vi "Script Cases.vi"(0 "primitive":i32, 1 "argument 1":dbl, 2 "argument 2":dbl, 3 "argument 3":dbl, 4 "argument 4":dbl, 5 "argument 5":dbl) -> ()   [LabVIEW 2014]
uses:
  Begin/Global Variables.vi
  Begin/Global RefNums.vi
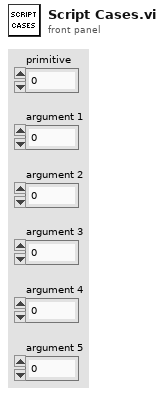
[diagram p1: front panel]
types:
  T1 = typedef "WPI_CounterDevRef.ctl" = cluster{"DevStatus":errorcluster, "CntIndex":T2}
  T2 = typedef "FPGA_CounterCtrSystemIndex.ctl" = enum8{"Ctr 0", "Ctr 1", "Ctr 2", "Ctr 3", "Ctr 4", "Ctr 5", "Ctr 6", "Ctr 7", "Invalid"}
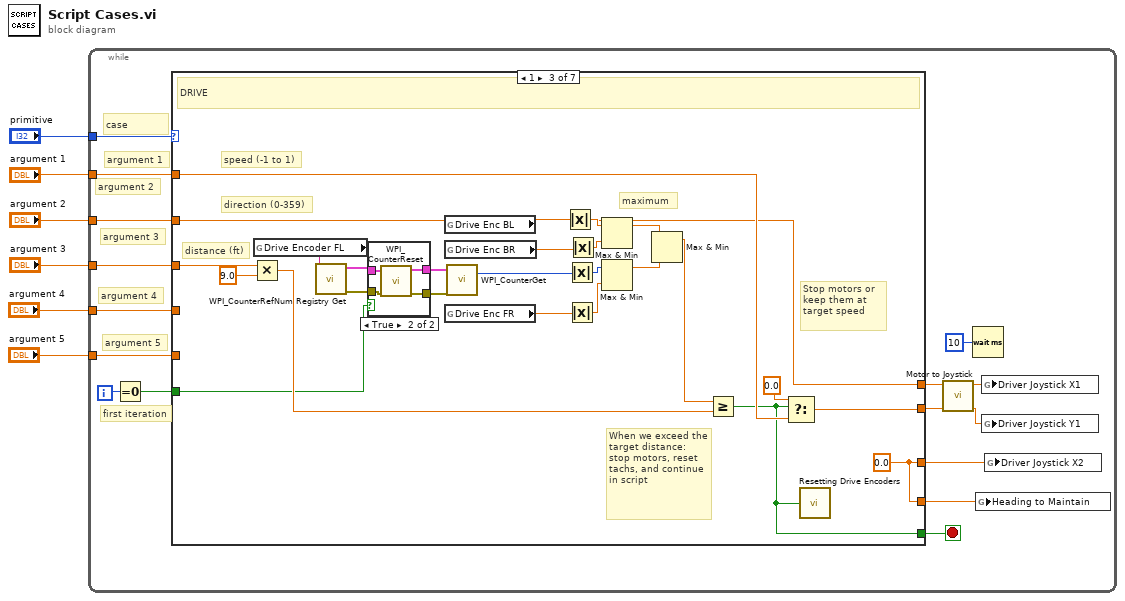
[diagram p0: block diagram]
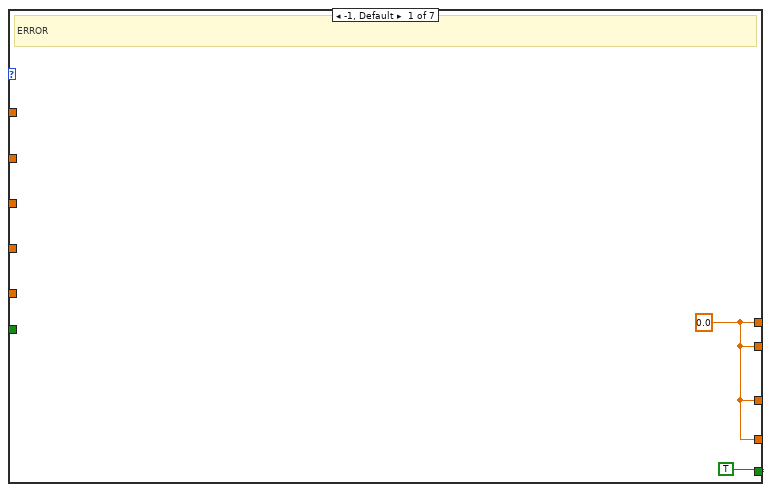
[diagram p2: hidden frame]
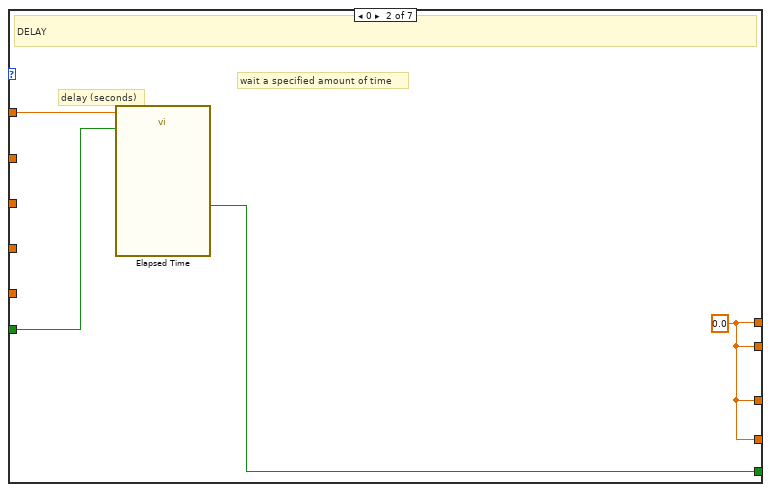
[diagram p3: hidden frame]
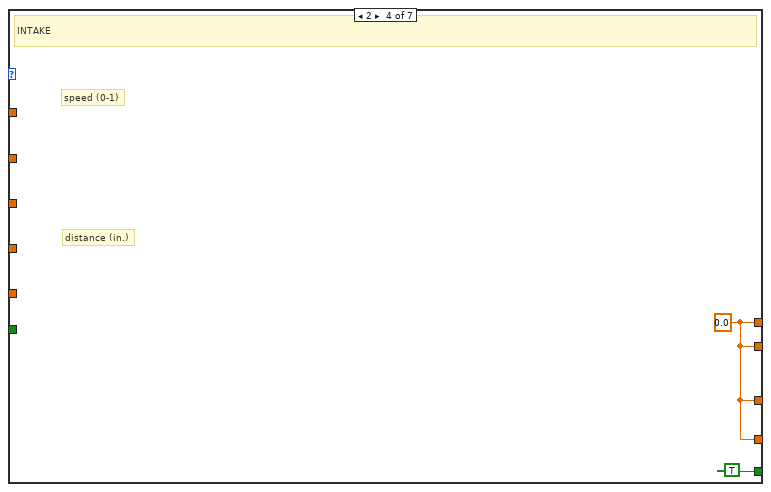
[diagram p5: hidden frame]
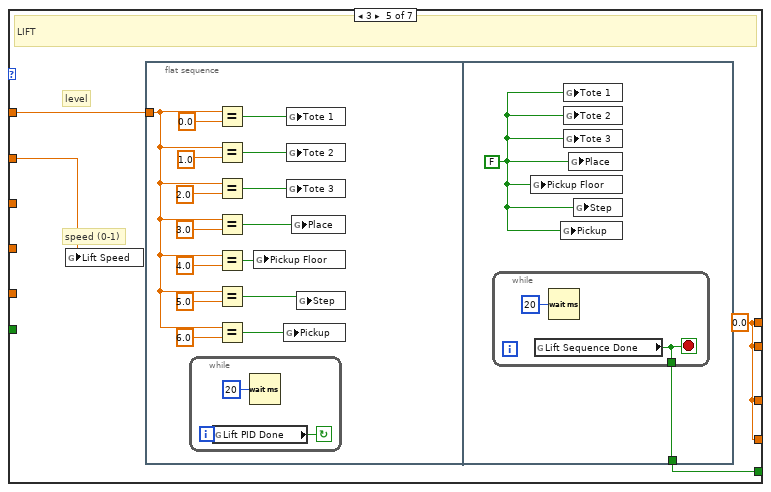
[diagram p6: hidden frame]
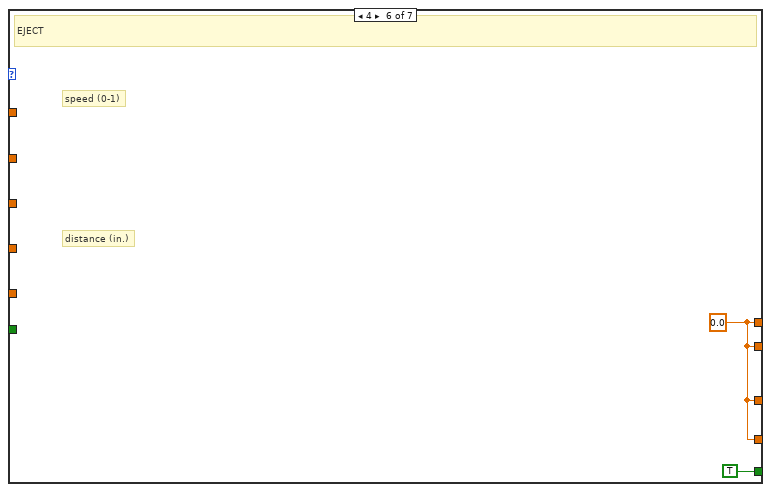
[diagram p7: hidden frame]
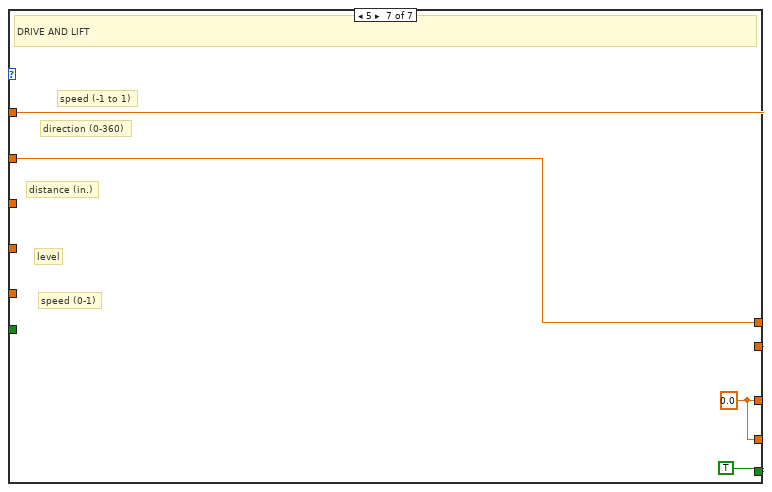
[diagram p8: hidden frame]
diagram:
  n1 = while {
    tunnel: "argument 1" -> [w22]
    tunnel: "argument 2" -> [w21]
    tunnel: "argument 3" -> [w20]
    tunnel: "argument 4" -> [w19]
    tunnel: "argument 5" -> [w18]
    tunnel: "primitive" -> [w17]
    i -> [w15]
    stop <- w16 stop-if-true
    # "first iteration"
    # "case"
    # "argument 5"
    # "argument 4"
    # "argument 3"
    # "argument 2"
    # "argument 1"
    n2 = Equal To 0?(x=w15) -> (x = 0?=w14:bool)
    n3 = case shown="1" w17 {
      tunnel: w22 -> [_ w28 w54 _ w65 _ w92]
      tunnel: w21 -> [_ _ w30 _ w66 _ w91]
      tunnel: w20 -> [_ _ w52 _ _ _ _]
      tunnel: w19 -> [_ _ _ _ _ _ _]
      tunnel: w18 -> [_ _ _ _ _ _ _]
      tunnel: [TRUE w26 w41 TRUE w63 TRUE TRUE] -> w16
      tunnel: w14 -> [_ w27 w34 _ _ _ _]
      tunnel: [w23 w25 w46 w61 w64 w88 w92] -> w11
      tunnel: [w23 w25 w30 w61 w64 w88 w91] -> w10
      tunnel: [w23 w25 w29 w61 w64 w88 w90] -> w9
      tunnel: [w23 w25 w29 w61 w64 w88 w90] -> w8
      frame -1, Default {
        w23 = 0.0 ("argument 1")
        # "ERROR"
      }
      frame 0 {
        w25 = 0.0 ("argument 1")
        # "wait a specified amount of time"
        # "delay (seconds)"
        # "DELAY"
        n4 = call "Elapsed Time"("Time Target (s)"=w28, "Reset"=w27) -> ("Time has Elapsed"=w26:bool)  [unwired: 10 in, 7 out]
      }
      frame 1 {
        w29 = 0.0 ("argument 1")
        # "When we exceed the target distance: stop motors, reset tachs, and continue in script"
        # "maximum"
        # "Stop motors or keep them at target speed"
        # "distance (ft)"
        # "direction (0-359)"
        # "speed (-1 to 1)"
        # "DRIVE"
        n5 = Multiply(x=w52, y=9.0) -> (x*y=w50:dbl)
        n6 = global read "Global RefNums.vi" "Drive Encoder FL"() -> (w35:string)
        n7 = call <vilib>:"WPI_CounterRefNum Registry Get.vi"("refnum name"=w35) -> ("error out"=w31:errorcluster, "CounterDevRef"=w32:T1)  [unwired: 9 in]
        n8 = case shown="True" w34 {
          tunnel: w32 -> [w56 w60]
          tunnel: w31 -> [w55 w59]
          tunnel: [w56 w58] -> w37
          tunnel: [w55 w57] -> w36
          frame False {
          }
          frame True {
            n9 = call <vilib>:"WPI_CounterReset.vi"("error in (no error)"=w59, "CounterDevRef in"=w60) -> ("error out"=w57:errorcluster, "CounterDevRef out"=w58:T1)  [unwired: 8 in]
          }
        }
        n10 = global read "Global Variables.vi" "Drive Enc BL"() -> (w40:dbl)
        n11 = global read "Global Variables.vi" "Drive Enc BR"() -> (w39:dbl)
        n12 = global read "Global Variables.vi" "Drive Enc FR"() -> (w38:dbl)
        n13 = call <vilib>:"WPI_CounterGet.vi"("error in (no error)"=w36, "CounterDevRef in"=w37) -> ("Value"=w33:i32)  [unwired: 4 in, 5 out]
        n14 = Absolute Value(x=w40) -> (abs(x)=w42:dbl)
        n15 = Absolute Value(x=w33) -> (abs(x)=w44:i32)
        n16 = Absolute Value(x=w38) -> (abs(x)=w43:dbl)
        n17 = Absolute Value(x=w39) -> (abs(x)=w45:dbl)
        n18 = Max & Min(x=w42, y=w45) -> (max(x,y)=w49:dbl)  [unwired: 1 out]
        n19 = Max & Min(x=w44, y=w43) -> (max(x,y)=w48:dbl)  [unwired: 1 out]
        n20 = Max & Min(x=w49, y=w48) -> (max(x,y)=w47:dbl)  [unwired: 1 out]
        n21 = Greater Or Equal?(x=w47, y=w50) -> (x >= y?=w41:bool)
        n22 = Select(t=0.0, s=w41, f=w54) -> (s? t:f=w46:dbl)
        n23 = call "Resetting Drive Encoders.vi"("Reset Encoders"=w41) -> ()  [unwired: 1 in]
      }
      frame 2 {
        w61 = 0.0 ("argument 1")
        # "distance (in.)"
        # "speed (0-1)"
        # "INTAKE"
      }
      frame 3 {
        w64 = 0.0 ("argument 1")
        # "speed (0-1)"
        # "level"
        # "LIFT"
        n24 = global write "Global Variables.vi" "Lift Speed"(w66) -> ()
        n25 = flat-sequence {
          tunnel: w65 -> [w68]
          tunnel: [w84] -> w63
          frame #0 {
            n26 = while {
              stop <- w82 continue-if-true
              n27 = global read "Global Variables.vi" "Lift PID Done"() -> (w82:bool)
              n28 = Wait (ms)(milliseconds to wait=u32 20) -> ()  [unwired: 1 out]
            }
            n29 = Equal?(x=w68, y=0.0 ("x")) -> (x = y?=w80:bool)
            n30 = Equal?(x=w68, y=1.0 ("x")) -> (x = y?=w79:bool)
            n31 = Equal?(x=w68, y=2.0 ("x")) -> (x = y?=w81:bool)
            n32 = Equal?(x=w68, y=3.0) -> (x = y?=w78:bool)
            n33 = Equal?(x=w68, y=4.0) -> (x = y?=w77:bool)
            n34 = Equal?(x=w68, y=5.0) -> (x = y?=w73:bool)
            n35 = Equal?(x=w68, y=6.0) -> (x = y?=w72:bool)
            n36 = global write "Global Variables.vi" "Pickup Floor"(w77) -> ()
            n37 = global write "Global Variables.vi" "Pickup"(w72) -> ()
            n38 = global write "Global Variables.vi" "Tote 1"(w80) -> ()
            n39 = global write "Global Variables.vi" "Tote 2"(w79) -> ()
            n40 = global write "Global Variables.vi" "Tote 3"(w81) -> ()
            n41 = global write "Global Variables.vi" "Place"(w78) -> ()
            n42 = global write "Global Variables.vi" "Step"(w73) -> ()
          }
          frame #1 {
            w85 = FALSE ("Tote 0")
            n43 = while {
              tunnel: [w86] -> w84
              stop <- w86 stop-if-true
              n44 = global read "Global Variables.vi" "Lift Sequence Done"() -> (w86:bool)
              n45 = Wait (ms)(milliseconds to wait=u32 20) -> ()  [unwired: 1 out]
            }
            n46 = global write "Global Variables.vi" "Pickup Floor"(w85) -> ()
            n47 = global write "Global Variables.vi" "Pickup"(w85) -> ()
            n48 = global write "Global Variables.vi" "Tote 1"(w85) -> ()
            n49 = global write "Global Variables.vi" "Tote 2"(w85) -> ()
            n50 = global write "Global Variables.vi" "Tote 3"(w85) -> ()
            n51 = global write "Global Variables.vi" "Place"(w85) -> ()
            n52 = global write "Global Variables.vi" "Step"(w85) -> ()
          }
        }
      }
      frame 4 {
        w88 = 0.0 ("argument 1")
        # "distance (in.)"
        # "speed (0-1)"
        # "EJECT"
      }
      frame 5 {
        w90 = 0.0 ("argument 1")
        # "speed (0-1)"
        # "level"
        # "distance (in.)"
        # "direction (0-360)"
        # "speed (-1 to 1)"
        # "DRIVE AND LIFT"
      }
    }
    n53 = call "Motor to Joystick.vi"("Drive Motor"=w11, "Rotational Motor"=w10) -> ("Joy Y"=w13:dbl, "Joy X"=w12:dbl)  [unwired: 8 in]
    n54 = Wait (ms)(milliseconds to wait=u32 10) -> ()  [unwired: 1 out]
    n55 = global write "Global Variables.vi" "Heading to Maintain"(w8) -> ()
    n56 = global write "Global Variables.vi" "Driver Joystick X1"(w12) -> ()
    n57 = global write "Global Variables.vi" "Driver Joystick Y1"(w13) -> ()
    n58 = global write "Global Variables.vi" "Driver Joystick X2"(w9) -> ()
  }
